vi "Toplevel_PolyStat.vi"() -> ()   [LabVIEW 2022 SP3]
doc: "This example performs writes and reads on a serial port, as directed by the user. You can press the Write and Read buttons, and change the Read Count, while the example is running.\n\nThe parameters set for the serial port must match the parameters of the connected instrument or device. In this example, the Read Count parameter specifies the number of bytes that the serial port reads. If there were more bytes at the port than the specified number, those bytes would not be read. If there were less bytes at the port than the specified number, you would receive a timeout error.\n\nThis example expands upon the flow control options for XON and XOFF, allowing the user to choose those control characters. Also, the user can enable or disable a termination character. Some devices require a termination character in order to identify the end of command strings. Some devices send a termination character to signify the end of data to be read. This example shows how you can end the Read operation once a termination character is detected in the buffer and/or append a termination character at the end of the Write data."
uses:
  Command_buttons.ctl
  Serial - Settings.ctl
  Serial - XON-XOFF Characters.ctl
  Serial - ASCII Characters.ctl
  fg_enum.ctl
  <vilib>/Instr/_visa.llb/VISA Configure Serial Port (Instr).vi
panel:
  out "Current\nTemp":dbl
  in  "Temperature\nto set":dbl
  in  "Stop":bool
  in  "Command Radio\nButtons":T1
  out "Response":string
  in  "Write":bool
  in  "Read":bool
  in  "VISA resource name":refnum<visa-resource-name>="COM1"
  # "------------------------\nPROGRAM EXECUTION   \n------------------------\n1. Connect PolyStat controller to PC via RS232 cable and choose corresponding port in 'VISA resource name'\n2. Set the time to poll which decides the time interval between each write-read pair or how often the command must be written and read\n3. Choose command to run by clicking the Radio buttons (can be changed during run). Refer the COMMANDS description for correct usage.\n4. Set the read and write buttons to ON for continuous polling mode\n5. Response can be observed on the given Response indicator\n6. Saved log PolyState_LabVIEW_log.txt can be found at LabVIEW default directory\n\nNOTE:\n> Only one command can be sent at a time\n> Program execution stops if controller response is negative\n> Program execution stops with error if no response is received from controller within 12 seconds after write\n> Time to poll cannot be changed during run, it is only read once at start"
  # "--------------\nCOMMANDS\n--------------\nP0 => Power off and standby\nP1 => Power on from standby\nF? => query fluid temperature\nS? => query current set temperature\nSn => set temperature to value n (change number between -40 to 105)\nValue of n should be given in 'Temperature to set' control\nUC => set unit to Celsius\nUF => set unit to Fahrenheit"
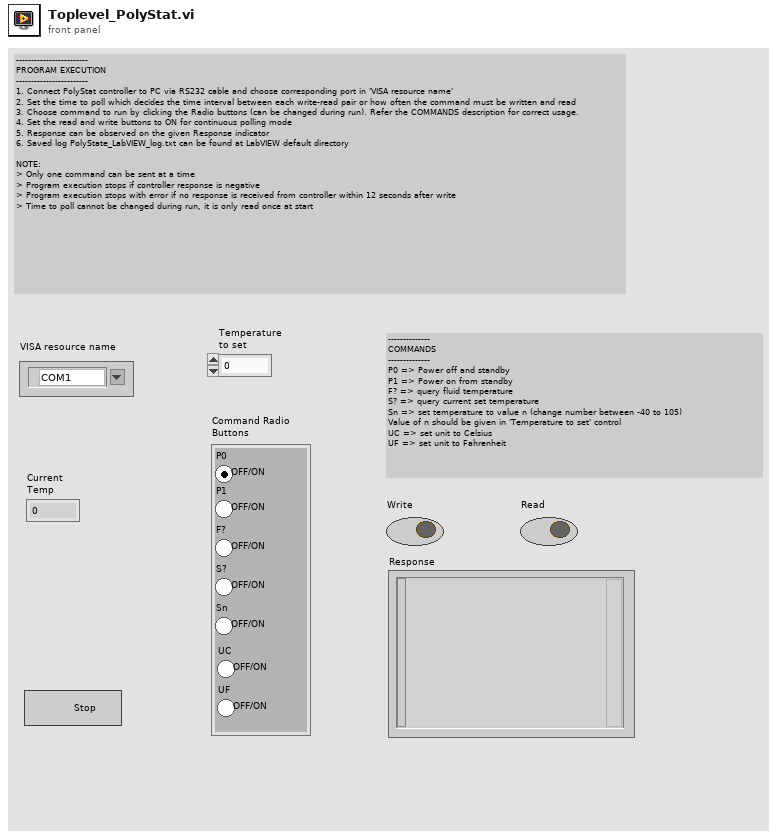
[diagram p1: front panel]
types:
  T1 = typedef "Command_buttons.ctl" = enum32{"P0", "P1", "F?", "S?", "Sn", "UC", "UF"}
  T2 = enum16{"open", "replace", "create", "open or create", "replace or create", "replace or create with confirmation"}
  T3 = typedef "Serial - XON-XOFF Characters.ctl" = cluster{"XON":T4, "XOFF":T4}
  T4 = typedef "Serial - ASCII Characters.ctl" = enum16{"NUL", "SOH", "STX", "ETX", "EOT", "ENQ", "ACK", "BEL", "BS", "HT", "LF", "VT", "FF", "CR", "SO", "SI", "DLE", "DC1", "DC2", "DC3", "DC4", "NAK", "SYN", "ETB", "CAN", "EM", "SUB", "ESC", "FS", "GS", "RS", "US", "SP", "!", "\"", "#", "$", "%", "&", "'", "(", ")", "*", "+", ",", "- (-)", ".", "/", "0", "1", "2", "3", "4", "5", "6", "7", "8", "9", ":", ";", "<", "=", ">", "?", "@", "A", "B", "C", "D", "E", "F", "G", "H", "I", "J", "K", "L", "M", "N", "O", "P", "Q", "R", "S", "T", "U", "V", "W", "X", "Y", "Z", "[", "\\", "]", "^", "_", "`", "a", "b", "c", "d", "e", "f", "g", "h", "i", "j", "k", "l", "m", "n", "o", "p", "q", "r", "s", "t", "u", "v", "w", "x", "y", "z", "{", "|", "}", "~"}
  T5 = typedef "Serial - Settings.ctl" = cluster{"baud rate":u32, "data bits":u16, "parity":enum16{"None", "Odd", "Even", "Mark", "Space"}, "stop bits":u16, "flow control":u16}
  T6 = typedef "fg_enum.ctl" = enum16{"SET", "RESET TIME", "GET"}
  T7 = typedef "Written_command.ctl" = string
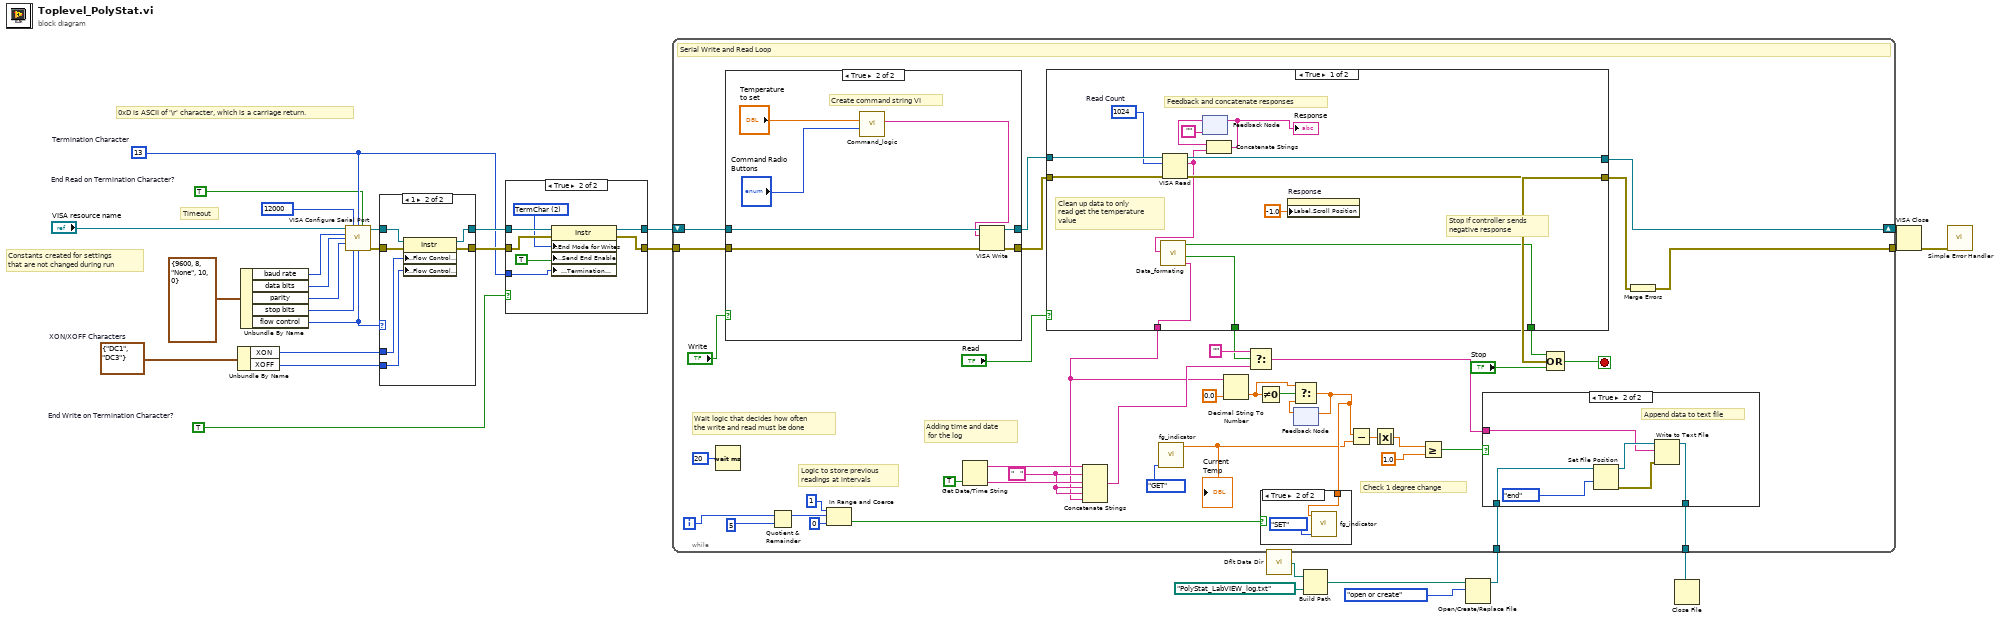
[diagram p0: block diagram]
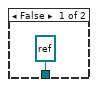
[diagram p5: hidden frame]
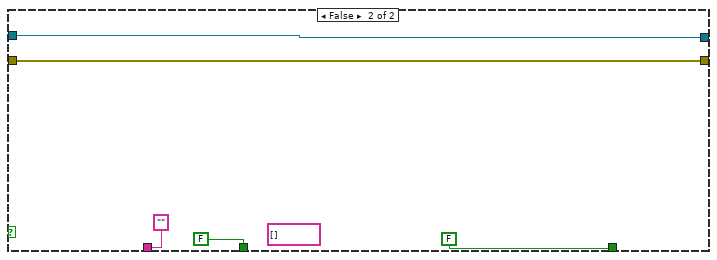
[diagram p7: hidden frame]
diagram:
  w8 = T3 {"XON"=enum."DC1", "XOFF"=enum."DC3"}  # XON/XOFF Characters
  w9 = TRUE  # End Write on Termination Character?
  w10 = TRUE  # End Read on Termination Character?
  w11 = u8 13  # Termination Character
  # "Constants created for settings\nthat are not changed during run"
  # "Timeout"
  # "0xD is ASCII of '\\r' character, which is a carriage return."
  n1 = Unbundle By Name(w8) -> ("XON"=w18:T4, "XOFF"=w17:T4)
  n2 = Unbundle By Name(T5 {"baud rate"=9600, "data bits"=8, "parity"=enum."None", "stop bits"=10, "flow control"=0} ("input cluster")) -> ("baud rate"=w23:u32, "data bits"=w24:u16, "parity"=w25:enum16{"None", "Odd", "Even", "Mark", "Space"}, "stop bits"=w26:u16, "flow control"=w19:u16)
  n3 = call-poly "VISA Configure Serial Port"("VISA resource name"="VISA resource name", "timeout (10sec)"=u32 12000, "termination char\n(0xA = '\\n' = LF)"=w11, "Enable Termination\nChar (T)"=w10, "baud rate (9600)"=w23, "data bits (8)"=w24, "parity (0:none)"=w25, "stop bits (10: 1 bit)"=w26, "flow control (0:none)"=w19) -> ("VISA resource name out"=w27:refnum<visa-resource-name>, "error out"=w28:errorcluster)  [unwired: 1 in, 4 out]
  n4 = case shown="1" w19 {
    tunnel: [w30 w37] -> w16
    tunnel: [w31 w36] -> w14
    tunnel: w28 -> [w30 w35]
    tunnel: w27 -> [w31 w34]
    tunnel: w18 -> [_ w33]
    tunnel: w17 -> [_ w32]
    frame Default {
    }
    frame 1 {
      n5 = property class="Instr"(reference=w34, error in=w35, "Serial Settings:Flow Control XON Character"=w33, "Serial Settings:Flow Control XOFF Character"=w32) -> (reference out=w36:refnum<visa-resource-name>, error out=w37:errorcluster)
    }
  }
  n6 = case shown="True" w9 {
    tunnel: w14 -> [w38 w46]
    tunnel: w16 -> [w39 w45]
    tunnel: [w38 w44] -> w13
    tunnel: [w39 w43] -> w15
    tunnel: w11 -> [_ w41]
    frame False {
    }
    frame True {
      w42 = u16 2 items=["None", "LastBit", "TermChar", "Break"] ("Serial Settings:Serial End Mode for Writes")
      n7 = property class="Instr"(reference=w46, error in=w45, "Serial Settings:End Mode for Writes"=w42, "Message Based Settings:Send End Enable"=TRUE, "Message Based Settings:Termination Character"=w41) -> (reference out=w44:refnum<visa-resource-name>, error out=w43:errorcluster)
    }
  }
  n8 = call <vilib>:"Dflt Data Dir.vi"() -> ("App:Default Data Directory"=w6:path)
  n9 = Build Path(base path=w6, name or relative path=path "PolyStat_LabVIEW_log.txt" ("default name")) -> (appended path=w3:path)
  n10 = Open/Create/Replace File(file path (use dialog)=w3, operation (0:open)=T2."open or create") -> (refnum out=w2:refnum<file>)  [unwired: 4 in, 2 out]
  n11 = while {
    shift-right: [w87] -> w20
    shift-left: w13 -> [w86]
    tunnel: w15 -> [w85]
    tunnel: [w76] -> w21
    tunnel: w2 -> [w68]
    tunnel: [w67] -> w1
    i -> [w65]
    stop <- w80 stop-if-true
    w50 = "   " ("string")
    # "Logic to store previous\nreadings at intervals"
    # "Check 1 degree change"
    # "Adding time and date\n for the log"
    # "Wait logic that decides how often\nthe write and read must be done"
    # "Serial Write and Read Loop"
    n12 = Wait (ms)(milliseconds to wait=u32 20) -> ()  [unwired: 1 out]
    n13 = case shown="True" "Write" {
      tunnel: w86 -> [w98 w105]
      tunnel: w85 -> [w97 w104]
      tunnel: [w98 w103] -> w79
      tunnel: [w97 w102] -> w84
      frame False {
      }
      frame True {
        # "Create command string VI"
        n14 = call "Command_logic.vi"("Command Radio Buttons"="Command Radio\nButtons", "Temperature\nto set"="Temperature\nto set") -> ("Written command"=w101:T7)  [unwired: 9 in]
        n15 = VISA Write(VISA resource name=w105, write buffer=w101, error in (no error)=w104) -> (VISA resource name out=w103:refnum<visa-resource-name>, error out=w102:errorcluster)  [unwired: 1 out]
      }
    }
    n16 = Quotient & Remainder(x=w65, y=5) -> (x-y*floor(x/y)=w64:i32)  [unwired: 1 out]
    n17 = In Range and Coerce(upper limit=1, x=w64, lower limit=0) -> (In Range?=w54:bool)  [unwired: 1 out]
    n18 = Get Date/Time String(want seconds? (F)=TRUE) -> (date string=w72:string, time string=w71:string)  [unwired: 2 in]
    n19 = case shown="True" "Read" {
      tunnel: [w116 w123] -> w87
      tunnel: w79 -> [w118 w123]
      tunnel: [w115 w122] -> w77
      tunnel: w84 -> [w117 w122]
      tunnel: [w108 ""] -> w47
      tunnel: [w109 FALSE] -> w81
      tunnel: [w110 FALSE] -> w74
      frame True {
        w112 = u32 1024  # Read Count
        # "Stop if controller sends\nnegative response"
        # "Clean up data to only\nread get the temperature\nvalue"
        # "Feedback and concatenate responses"
        n20 = VISA Read(VISA resource name=w118, byte count=w112, error in (no error)=w117) -> (VISA resource name out=w116:refnum<visa-resource-name>, read buffer=w111:string, error out=w115:errorcluster)  [unwired: 1 out]
        n21 = call "Data_formating.vi"("String"=w111) -> ("Result string"=w108:string, "Space not found?"=w110:bool, "Negative response?"=w109:bool)  [unwired: 7 in, 1 out]
        n22 = feedback #1("") -> (w114:string)
        n23 = Concatenate Strings(w114, w111) -> (w107:string)
        "Response" <- w107
        n24 = feedback-in #1(w107) -> ()
        n25 = property on="Response" class="Str"("Label.Scroll Position"=-1.0) -> ()  [unwired: 2 in, 2 out]
      }
      frame False {
        (unwired) string[] []
      }
    }
    n26 = Concatenate Strings(w72, w50, w71, w50, w50, w47) -> (w70:string)
    n27 = call "fg_indicator.vi"("Mode selector"=fg_enum."GET") -> ("Output"=w48:dbl)  [unwired: 8 in, 2 out]
    "Current\nTemp" <- w48
    n28 = Decimal String To Number(string=w47, default (0L)=0.0 ("default (0 I32)")) -> (number=w56:dbl)  [unwired: 1 in, 1 out]
    n29 = Select(t="", s=w74, f=w70) -> (s? t:f=w63:string)
    n30 = Not Equal To 0?(x=w56) -> (x != 0?=w57:bool)
    n31 = feedback #2() -> (w55:dbl)  [unwired: 1 in]
    n32 = Select(t=w56, s=w57, f=w55) -> (s? t:f=w53:dbl)
    n33 = case shown="True" w54 {
      tunnel: w53 -> [_ w88]
      frame False {
      }
      frame True {
        n34 = call "fg_indicator.vi"("Mode selector"=fg_enum."SET", "Numeric"=w88) -> ()  [unwired: 7 in, 3 out]
      }
    }
    n35 = feedback-in #2(w53) -> ()
    n36 = Subtract(x=w53, y=w48) -> (x-y=w59:dbl)
    n37 = Absolute Value(x=w59) -> (abs(x)=w58:dbl)
    n38 = Greater Or Equal?(x=w58, y=1.0) -> (x >= y?=w52:bool)
    n39 = case shown="True" w52 {
      tunnel: w68 -> [_ w93]
      tunnel: [refnum<file> refnum ("refnum out") w92] -> w67
      tunnel: w63 -> [_ w91]
      frame False {
      }
      frame True {
        # "Append data to text file"
        n40 = Set File Position(refnum=w93, from (0:start)=enum16{"start", "end", "current"}."end") -> (refnum out=w95:refnum<file>, error out=w96:errorcluster)  [unwired: 2 in]
        n41 = Write to Text File(file (use dialog)=w95, text=w91, error in=w96) -> (refnum out=w92:refnum<file>)  [unwired: 1 in, 2 out]
      }
    }
    n42 = Compound Arithmetic op=OR(w81, w77, "Stop") -> (w80:bool)
    n43 = Merge Errors(w77) -> (w76:errorcluster)
  }
  n44 = Close File(refnum=w1) -> ()  [unwired: 1 in, 2 out]
  n45 = VISA Close(VISA resource name=w20, error in (no error)=w21) -> (error out=w22:errorcluster)
  n46 = call <vilib>:"Simple Error Handler.vi"("error in (no error)"=w22) -> ()  [unwired: 1 in, 8 out]
